vi "LabView360-条件结构.vi"() -> ()   [LabVIEW 2018]
panel:
  out "输出变量":dbl
  in  "数值":dbl
  out "字符串 2":string
  in  "字符串":string
  in  "布尔":bool
  in  "确定按钮":bool
  out "result":dbl
  in  "B":dbl
  in  "A":dbl
  in  "s":bool
  out "s? t:f":dbl
  # "A-B"
  # "A+B"
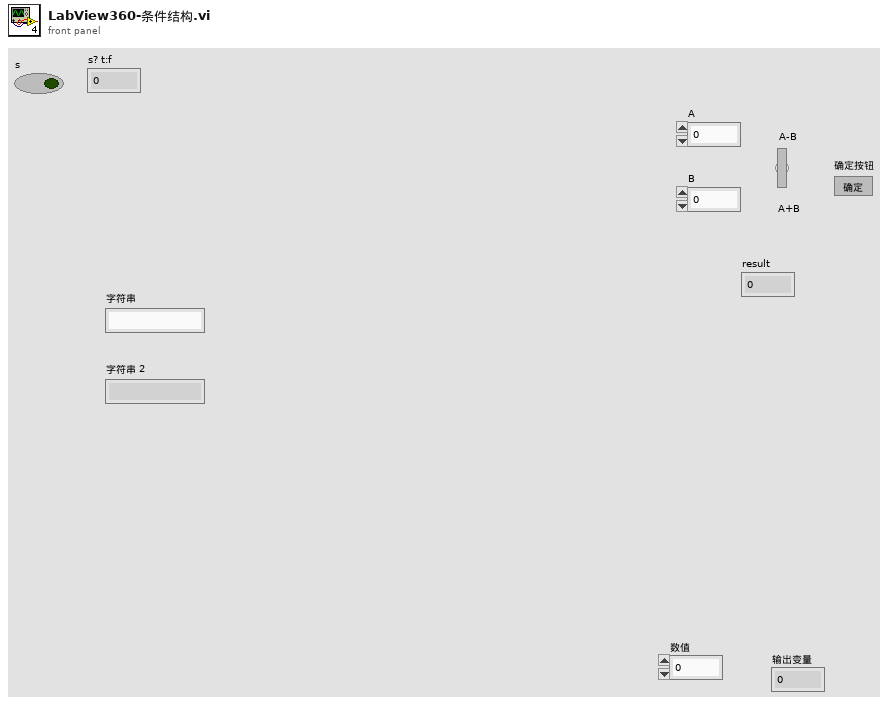
[diagram p1: front panel]
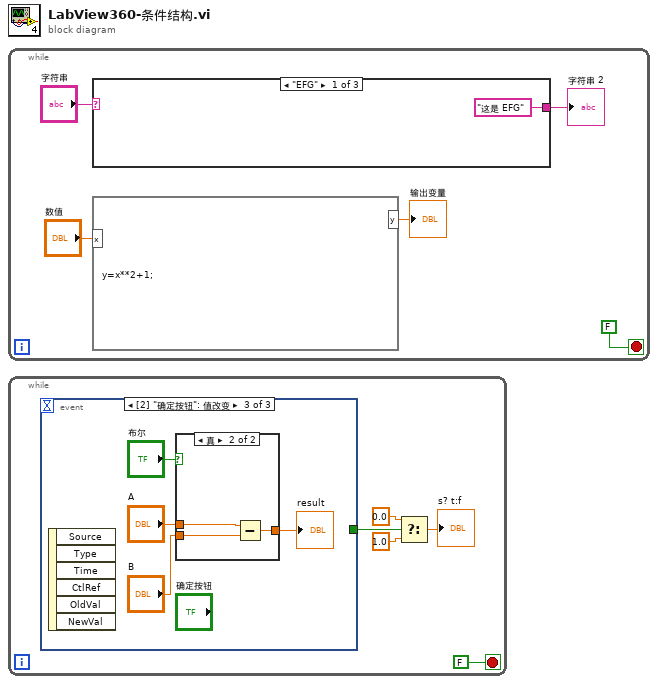
[diagram p0: block diagram]
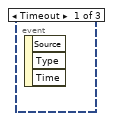
[diagram p2: hidden frame]
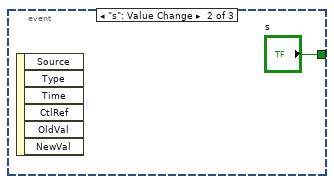
[diagram p3: hidden frame]
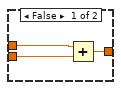
[diagram p4: hidden frame]
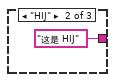
[diagram p5: hidden frame]
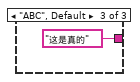
[diagram p6: hidden frame]
diagram:
  n1 = while {
    stop <- FALSE stop-if-true
    n2 = case shown="\"EFG\"" "字符串" {
      tunnel: ["这是 EFG" "这是 HIJ" "这是真的"] -> w3
      frame "EFG" {
      }
      frame "HIJ" {
      }
      frame "ABC", Default {
      }
    }
    "字符串 2" <- w3
    n3 = formula code="y=x**2+1;"("x"="数值") -> ("y"=→"输出变量":dbl)
  }
  n4 = while {
    stop <- FALSE stop-if-true
    n5 = event shown="[2] \"确定按钮\": 值改变" {
      selector: _ -> [_ _ _]
      dyn-events: _ -> [_ _ _]
      timeout: _ -> [_ _ _]
      tunnel: [_ "s" _] -> w13
      event Timeout {
        n6 = event-data() -> ()  [unwired: 1 in, 3 out]
      }
      event "s": Value Change {
        n7 = event-data() -> ()  [unwired: 1 in, 6 out]
      }
      event "确定按钮": Value Change {
        n8 = event-data() -> ()  [unwired: 1 in, 6 out]
        n9 = case shown="真" "布尔" {
          tunnel: "A" -> [w21 w24]
          tunnel: "B" -> [w20 w23]
          tunnel: [w19 w22] -> w16
          frame False {
            n10 = Add(x=w21, y=w20) -> (x+y=w19:dbl)
          }
          frame True {
            n11 = Subtract(x=w24, y=w23) -> (x-y=w22:dbl)
          }
        }
        "result" <- w16
      }
    }
    n12 = Select(t=0.0, s=w13, f=1.0) -> (s? t:f=→"s? t:f":dbl)
  }
